vi "DAXSetTGC.vi"(7 "Daxsonics Name":T1, 8 "error IN":errorcluster, 9 "TGC Times":cluster{dbl, dbl}, 11 "VISA resource name":refnum<visa-resource-name>="ASRL4::INSTR") -> (0 "error out":errorcluster)   [LabVIEW 2022 SP3]
uses:
  Daxsonics_Pulsers.ctl
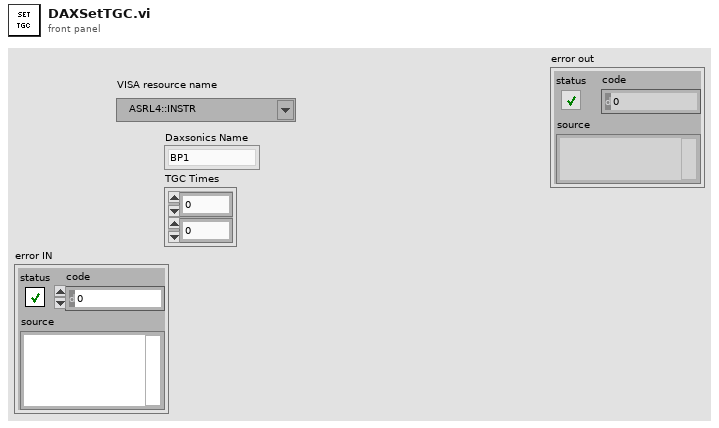
[diagram p1: front panel]
types:
  T1 = typedef "Daxsonics_Pulsers.ctl" = enum16{"BP1", "BP2_A", "BP2_B", "10ERS8", "New2021"}
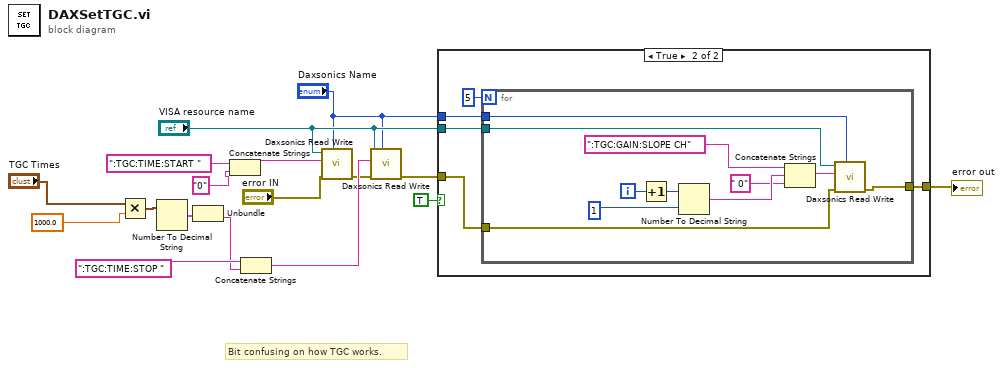
[diagram p0: block diagram]
diagram:
  # "Bit confusing on how TGC works."
  n1 = Multiply(x="TGC Times", y=1000.0) -> (x*y=w14:cluster{dbl, dbl})
  n2 = Number To Decimal String(number=w14) -> (decimal integer string=w13:cluster{string, string})  [unwired: 1 in]
  n3 = Unbundle(w13) -> (w2:string)  [unwired: 1 out]
  n4 = Concatenate Strings(":TGC:TIME:START " ("string"), "0") -> (w12:string)
  n5 = Concatenate Strings(":TGC:TIME:STOP " ("string"), w2) -> (w11:string)
  n6 = call "Daxsonics Read Write.vi"("Daxsonics Name"="Daxsonics Name", "error IN"="error IN", "write buffer"=w12, "VISA resource name"="VISA resource name") -> ("error out"=w10:errorcluster)  [unwired: 5 in, 2 out]
  n7 = call "Daxsonics Read Write.vi"("Daxsonics Name"="Daxsonics Name", "error IN"=w10, "write buffer"=w11, "VISA resource name"="VISA resource name") -> ("error out"=w9:errorcluster)  [unwired: 5 in, 2 out]
  n8 = case shown="True" TRUE {
    tunnel: w9 -> [w18 w22]
    tunnel: "VISA resource name" -> [_ w21]
    tunnel: "Daxsonics Name" -> [_ w20]
    tunnel: [w18 w19] -> w4
    frame False {
    }
    frame True {
      n9 = for {
        N: 5 -> [_]
        tunnel: w22 -> [w27]
        tunnel: w21 -> [w26]
        tunnel: w20 -> [w25]
        tunnel: [w24] -> w19
        i -> [w34]
        n10 = Increment(x=w34) -> (x+1=w32:i32)
        n11 = Number To Decimal String(number=w32, width (-)=1) -> (decimal integer string=w33:string)
        n12 = Concatenate Strings(":TGC:GAIN:SLOPE CH" ("string"), w33, " 0") -> (w28:string)
        n13 = call "Daxsonics Read Write.vi"("Daxsonics Name"=w25, "error IN"=w27, "write buffer"=w28, "VISA resource name"=w26) -> ("error out"=w24:errorcluster)  [unwired: 5 in, 2 out]
      }
    }
  }
  "error out" <- w4
